vi "Passing Paramters Complex Struct.vi"(7 "y":i32, 8 "error in (no error)":errorcluster, 9 "x":i32, 10 "numVertices":i32, 11 "name":u32) -> (0 "error out":errorcluster, 3 "function return":i32)   [LabVIEW 2009, in "LabVIEWWrapper_PassingDataSampleDLL.lvlib"]
doc: "int PassingParamters_ComplexStruct (struct complexStructPolygon triangle);"
uses:
  LabVIEWWrapper_PassingDataSampleDLL.lvlib
  PassingDataSampleDLL.dll
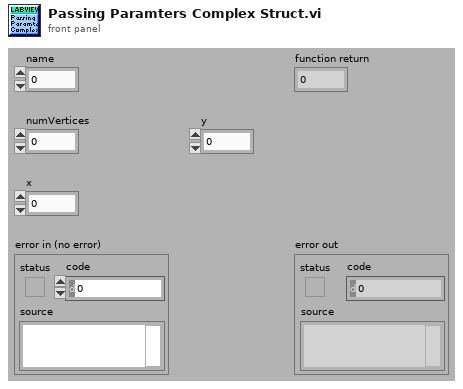
[diagram p1: front panel]
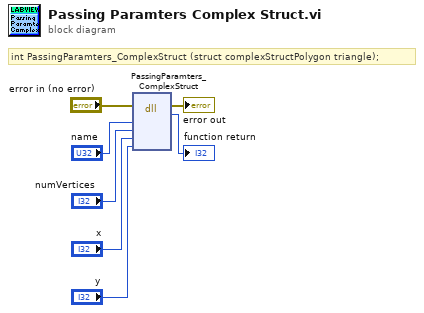
[diagram p0: block diagram]
diagram:
  # "int PassingParamters_ComplexStruct (struct complexStructPolygon triangle);"
  n1 = dll-call lib="C:/My Dropbox/Systems Engineering Application/SDK/C Integration/LabVIEWWrapper/PassingDataSampleDLL.*" fn="PassingParamters_ComplexStruct"(error in="error in (no error)", "name"="name", "numVertices"="numVertices", "x"="x", "y"="y") -> (error out=→"error out":errorcluster, →"function return":i32)  [unwired: 6 in, 1 out]
